vi "Create Host Stream Refs.vi"(8 "error in (no error)":errorcluster, 10 "Addon":string, 11 "Target IP Address":string) -> (0 "error out":errorcluster, 3 "Refs":T1)   [LabVIEW 2019, in "CAN Stream Support Workspace Shared.lvlib"]
uses:
  CAN Stream Support Workspace Shared.lvlib
  Types/Host Stream Refs.ctl
  <vilib>/xnet/xnet.llb/XNET CAN Comm.ctl
  <vilib>/xnet/xnet.llb/XNET CAN Comm State.ctl
  <vilib>/xnet/xnet.llb/XNET CAN Last Err.ctl
  <vilib>/xnet/xnet.llb/XNET Frame CAN.ctl
  <vilib>/xnet/xnet.llb/XNET Frame Type CAN.ctl
  Addon/Addon Shared/Types/Stream Type.ctl
  Addon/Addon Shared/CAN Stream Support Shared.lvlib
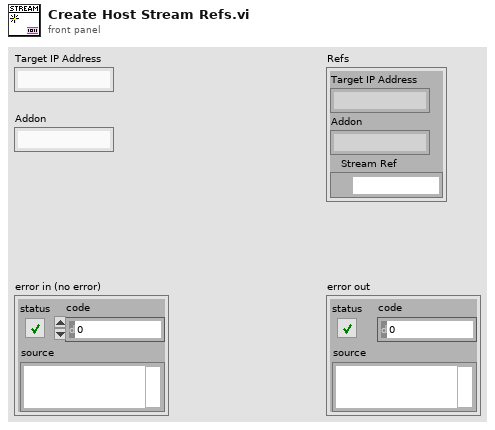
[diagram p1: front panel]
types:
  T1 = typedef "CAN Stream Support Workspace Shared.lvlib/Host Stream Refs.ctl" = cluster{"Target IP Address":string, "Addon":string, "Stream Ref":refnum<k21>}
  T2 = typedef "CAN Stream Support Shared.lvlib/Stream Type.ctl" = cluster{"State":T3, "Frames":T6[]}
  T3 = typedef "XNET CAN Comm.ctl" = cluster{"fault code":i32, "fault?":bool, "communication state":T4, "last error":T5, "receive error counter":u8, "transmit error counter":u8, "transceiver error?":bool, "sleep?":bool}
  T4 = typedef "XNET CAN Comm State.ctl" = u8
  T5 = typedef "XNET CAN Last Err.ctl" = u8
  T6 = typedef "XNET Frame CAN.ctl" = cluster{"timestamp":timestamp, "payload":u8[], "identifier":u32, "type":T7, "extended?":bool, "echo?":bool}
  T7 = typedef "XNET Frame Type CAN.ctl" = u8
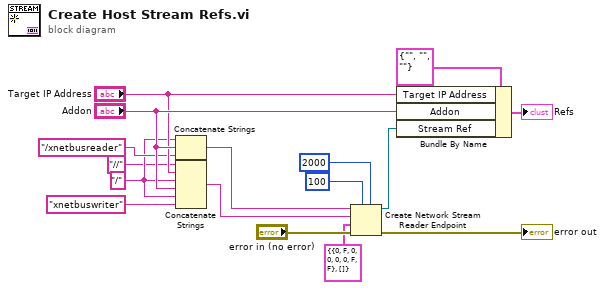
[diagram p0: block diagram]
diagram:
  w9 = "/" ("string")
  n1 = Concatenate Strings(w9, "Addon", "/xnetbusreader" ("writer name")) -> (w11:string)
  n2 = Concatenate Strings("//" ("reader url"), "Target IP Address", w9, "Addon", w9, "xnetbuswriter" ("reader url")) -> (w8:string)
  n3 = Create Network Stream Reader Endpoint(5:2000 ("timeout in ms (-1)"), 7:100 ("reader buffer size"), 8:"error in (no error)", 9:T2 {"State"={"fault code"=0, "fault?"=FALSE, "communication state"=0, "last error"=0, "receive error counter"=0, "transmit error counter"=0, "transceiver error?"=FALSE, "sleep?"=FALSE}, "Frames"=[]} ("Stream"), 10:w8, 11:w11) -> (0:→"error out":errorcluster, 3:w2:refnum<k21>)  [unwired: 1 in]
  n4 = Bundle By Name(cluster=T1 {"Target IP Address"="", "Addon"="", "Stream Ref"=""}, "Target IP Address"="Target IP Address", "Addon"="Addon", "Stream Ref"=w2) -> (→"Refs":T1)
